vi "Store Position.vi"(8 "error in (no error)":errorcluster, 10 "Position Message":T1, 11 "GUI Manager Module in":refnum<class "GUI Manager Module.lvclass">) -> (0 "error out":errorcluster, 3 "GUI Manager Module out":refnum<class "GUI Manager Module.lvclass">)   [LabVIEW 2020, in "VolatusGUI.lvlib" / "GUI Manager Module.lvclass"]
uses:
  GUI Manager Module.lvclass
  Position Data.ctl
  <vilib>/Utility/miscctls.llb/LVRectTypeDef.ctl
  GUI Manager Module.lvclass/GUI Manager Module.ctl
  lv-userprefs/User Prefs/Pref Group/Pref Group.lvclass
  VolatusGUI.lvlib
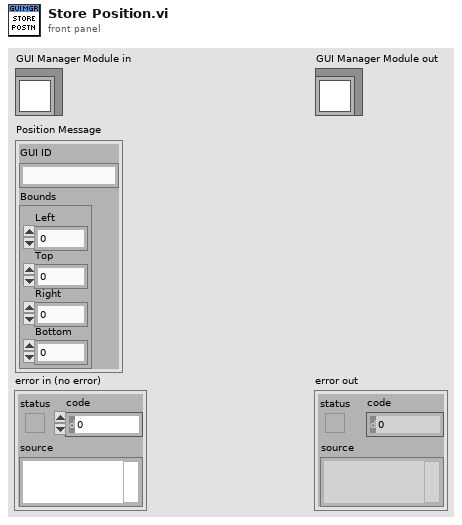
[diagram p1: front panel]
types:
  T1 = typedef "VolatusGUI.lvlib/Position Data.ctl" = cluster{"GUI ID":string, "Bounds":T2}
  T2 = typedef "LVRectTypeDef.ctl" = cluster{"Left":i16, "Top":i16, "Right":i16, "Bottom":i16}
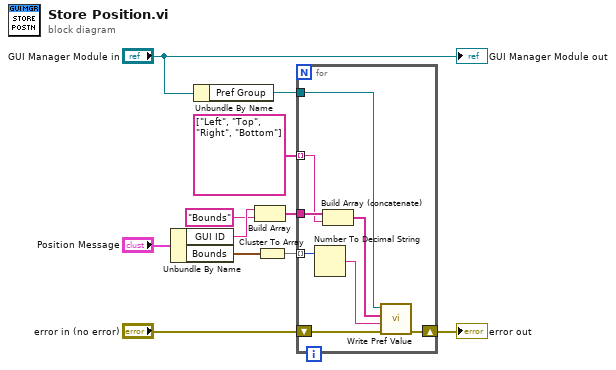
[diagram p0: block diagram]
diagram:
  n1 = Unbundle By Name("Position Message") -> ("GUI ID"=w7:string, "Bounds"=w10:T2)
  n2 = Unbundle By Name("GUI Manager Module in") -> ("Pref Group"=w3:refnum<class "Pref Group.lvclass">)
  n3 = Build Array(w7, "Bounds" ("element")) -> (w5:string[])
  n4 = Cluster To Array(cluster=w10) -> (array=w9:i16[])
  n5 = for {
    tunnel: w9 -> [w18] mode=indexing
    tunnel: string[] ["Left", "Top", "Right", "Bottom"] -> [w15] mode=indexing
    tunnel: w5 -> [w16]
    tunnel: w3 -> [w19]
    shift-right: [w13] -> w2
    shift-left: "error in (no error)" -> [w12]
    n6 = Number To Decimal String(number=w18) -> (decimal integer string=w17:string)  [unwired: 1 in]
    n7 = Build Array (concatenate)(w16, w15) -> (w14:string[])
    n8 = call "Write Pref Value.vi"("error in (no error)"=w12, "Value"=w17, "Pref Hierarchy"=w14, "Pref Group in"=w19) -> ("error out"=w13:errorcluster)  [unwired: 6 in, 1 out]
  }
  "error out" <- w2
  "GUI Manager Module out" <- "GUI Manager Module in"
